vi "Check.vi"(4 "Encoding":T2=32 items=["Raw"=32, "Base64"=64], 6 "Type":T3=1 items=["Plain"=1, "SHA1"=2, "Custom"=3], 7 "Port":i32=22, 8 "Error In":errorcluster, 9 "Host Key":u8[](array[numeric]), 10 "Address":string, 11 "KnownHosts In":refnum<class "Known Hosts.lvclass">) -> (0 "Error Out":errorcluster, 2 "Result":T1 items=["Match", "Mismatch", "Not Found", "Failure"], 3 "KnownHosts Out":refnum<class "Known Hosts.lvclass">)   [LabVIEW 2018, in "Toolkit.lvlib" / "Known Hosts.lvclass"]
uses:
  Known Hosts.lvclass
  Type Definitions/Host Name Types.ctl
  Type Definitions/Key Encodings.ctl
  Type Definitions/Check Results.ctl
  Known Hosts.lvclass/Known Hosts.ctl
  Session/Session.lvclass/Session.ctl
  SSH/SSH.lvclass/SSH.ctl
  Toolkit.lvlib
  Session/Session.lvclass
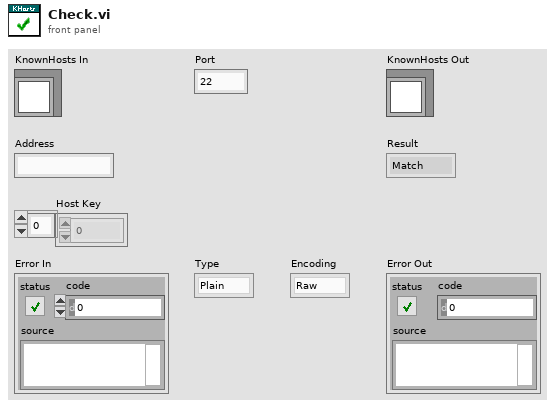
[diagram p1: front panel]
types:
  T1 = typedef "Toolkit.lvlib/Known Hosts.lvclass/Check Results.ctl" = i32
  T2 = typedef "Toolkit.lvlib/Known Hosts.lvclass/Key Encodings.ctl" = i32
  T3 = typedef "Toolkit.lvlib/Known Hosts.lvclass/Host Name Types.ctl" = i32
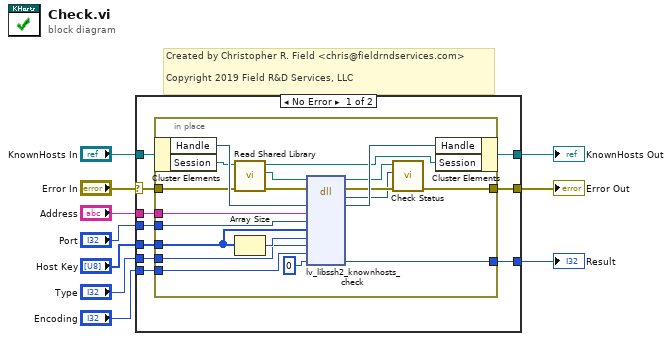
[diagram p0: block diagram]
diagram:
  # "Created by Christopher R. Field <chris@fieldrndservices.com>\n\nCopyright 2019 Field R&D Services, LLC"
  n1 = case shown="No Error" "Error In" {
    selector: "Error In" -> [w18 w41]
    tunnel: "KnownHosts In" -> [w20 w40]
    tunnel: [w17 w41] -> w8
    tunnel: [w19 w40] -> w7
    tunnel: "Address" -> [w16 _]
    tunnel: "Host Key" -> [w15 _]
    tunnel: "Type" -> [w14 _]
    tunnel: "Encoding" -> [w13 _]
    tunnel: "Port" -> [w12 _]
    tunnel: [w11 _] -> w1
    frame No Error {
      n2 = in-place {
        in-place-border: w18 -> [w34]
        in-place-border: [w33] -> w17
        in-place-border: w16 -> [w35]
        in-place-border: w15 -> [w30]
        in-place-border: w14 -> [w22]
        in-place-border: w13 -> [w21]
        in-place-border: w12 -> [w31]
        in-place-border: [w23] -> w11
        n3 = in-place-cluster #1(w20) -> ("Handle"=w39:u64, "Session"=w26:refnum<class "Session.lvclass">)
        n4 = call "Read Shared Library.vi"("Error In"=w34, "Session In"=w26) -> ("Erorr Out"=w27:errorcluster, "libssh2lv Shared Library"=w25:path, "Session Out"=w24:refnum<class "Session.lvclass">)  [unwired: 7 in]
        n5 = Array Size(array=w30) -> (size(s)=w29:i32)
        n6 = dll-call lib="D:/Users/cfield/Code/Field R&D Services/SSH/LV-LIBSSH2/LabVIEW/trunk/src/Toolkit/Support/lv-libssh2.*" fn="lv_libssh2_knownhosts_check"(path in=w25, error in=w27, "handle"=w39, "host"=w35, "port"=w31, "host_key"=w30, "host_key_len"=w29, "type"=w22, "encoding"=w21, "result"=0) -> (path out=w36:path, error out=w37:errorcluster, "status"=w32:i32, "handle"=w38:u64, "result"=w23:i32)  [unwired: 7 in]
        n7 = call "Check Status.vi"("Error In"=w37, "Status"=w32, "lv-libssh2 Shared Library In"=w36) -> ("Error Out"=w33:errorcluster)  [unwired: 7 in, 1 out]
        n8 = in-place-cluster #1("Handle"=w38, "Session"=w24) -> (w19:refnum<class "Known Hosts.lvclass">)
      }
    }
    frame Error {
    }
  }
  "Error Out" <- w8
  "KnownHosts Out" <- w7
  "Result" <- w1
